vi "Step Abort Action.vi"(8 "error in (no error)":errorcluster, 10 "Step":refnum<class "Step.lvclass">, 11 "Tester in":refnum<class "Tester.lvclass">) -> (0 "error out":errorcluster, 3 "Tester out":refnum<class "Tester.lvclass">)   [LabVIEW 2020, in "Tester.lvlib" / "Tester.lvclass"]
uses:
  Tester.lvclass
  Step/Step.lvclass
  Results/Result.ctl
  Results/Results.lvclass
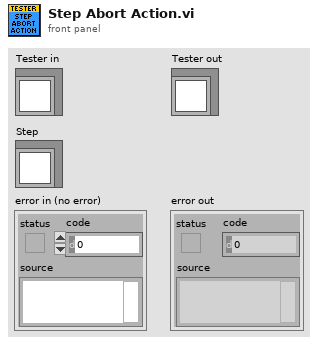
[diagram p1: front panel]
types:
  T1 = typedef "Tester.lvlib/Results.lvclass/Result.ctl" = enum16{"No Result", "Pass", "Fail", "Error", "Abort"}
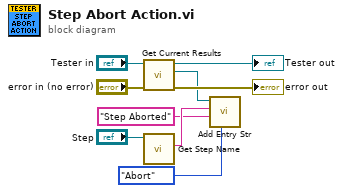
[diagram p0: block diagram]
diagram:
  n1 = call "Get Current Results.vi"("error in (no error)"="error in (no error)", "Tester in"="Tester in") -> ("error out"=→"error out":errorcluster, "Current Results"=w5:refnum<class "Results.lvclass">, "Tester out"=→"Tester out":refnum<class "Tester.lvclass">)  [unwired: 7 in]
  n2 = call-dynamic "Get Step Name.vi"("Step in"="Step") -> ("Step Name"=w2:string)  [unwired: 8 in, 2 out]
  n3 = call "Add Entry Str.vi"("Result"=Result."Abort", "Value Str"="Step Aborted" ("Name"), "Name"=w2, "Results in"=w5) -> ()  [unwired: 6 in, 2 out]
